vi "Draw.vi"(8 "error in (no error)":errorcluster, 11 "Terminal in":refnum<class "Terminal.lvclass">) -> (0 "error out":errorcluster, 2 "Picture":picture, 3 "Terminal out":refnum<class "Terminal.lvclass">)   [LabVIEW 2015, in "Terminal.lvclass"]
uses:
  Terminal.lvclass
  Concatenated Shape/Concatenated Shape.lvclass
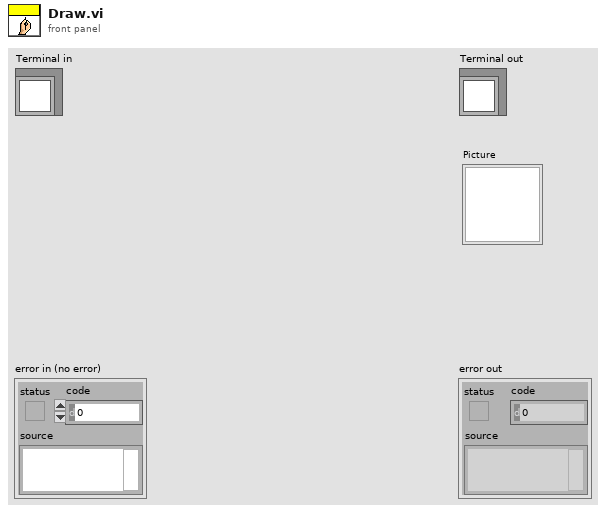
[diagram p1: front panel]
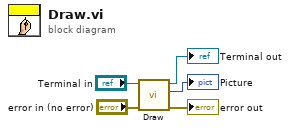
[diagram p0: block diagram]
diagram:
  n1 = call-parent "Draw.vi"("error in (no error)"="error in (no error)", "Concatenated Shape in"="Terminal in") -> ("error out"=→"error out":errorcluster, "Picture"=→"Picture":picture, "Concatenated Shape out"=→"Terminal out":refnum<class "Terminal.lvclass">)  [unwired: 7 in]
